vi "SUMMER SUNDAY BYTE[6].vi"() -> ()   [LabVIEW 2009]
uses:
  <vilib>/ULx/Create Channel.llb/ULx Create Channel (AI-Voltage-Basic).vi
  <vilib>/ULx/Create Channel.llb/ULx Create Channel (DO-Digital Output).vi
  <vilib>/ULx/Create Channel.llb/ULx Create Channel (DI-Digital Input).vi
  <vilib>/ULx/Write.llb/ULx Write (Digital Bool 1Line 1Point).vi
  <vilib>/ULx/Read.llb/ULx Read (Analog DBL 1Chan 1Samp).vi
  <vilib>/ULx/Read.llb/ULx Read (Digital 1D U8 NChan 1Samp).vi
  <vilib>/ULx/Read.llb/ULx Read (Digital Bool 1Line 1Point).vi
panel:
  out "BitValue":bool
  out "max value":u8
  out "POWER":bool
  out "data":dbl format="%_6g"
  out "ENERGY LEVEL":dbl(knob) scale=0.0..15.0
  out "Beam Pot":dbl format="%_6g"
  out "READY 2":bool
  out "DUMP":bool
  out "POWER":bool
  out "?":bool
  out "?":bool
  out "?":bool
  out "?":bool
  out "?":bool
  out "?":bool
  out "?":bool
  out "?":bool
  out "?":bool
  out "?":bool
  out "OPEN":bool
  out "CLOSED":bool
  out "READY":bool
  out "FAULT":bool
  out "MAGNET FORCE":dbl(slide) scale=0.0..10.0
  out "READY":bool
  out "TEMPERATURE":dbl(slide) scale=0.0..100.0
  in  "stop":bool
  out "?":bool
  out "?":bool
  out "?":bool
  out "?":bool
  out "FAULT":bool
  out "POWER":bool
  out "FLOW IN GPM":dbl(knob) scale=0.0..15.0
  # "USERS LAB AREA"
  # "BEAM STATUS"
  # "ROOM"
  # "XRAY"
  # "PUMP STATION"
  # "MAGNET STATUS"
  # "ORBIT"
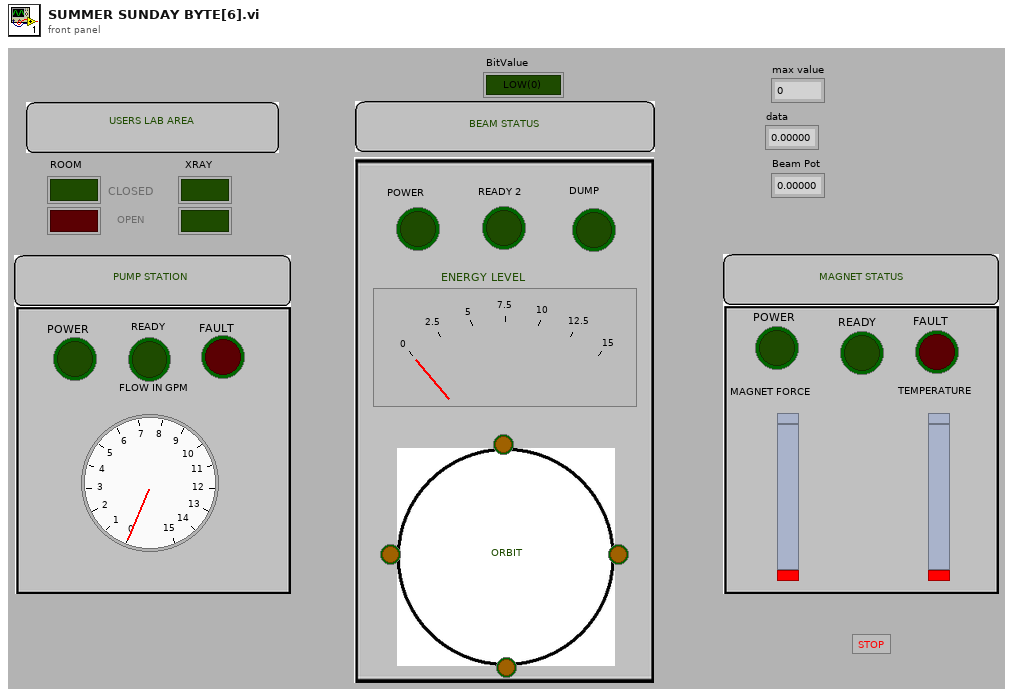
[diagram p1: front panel]
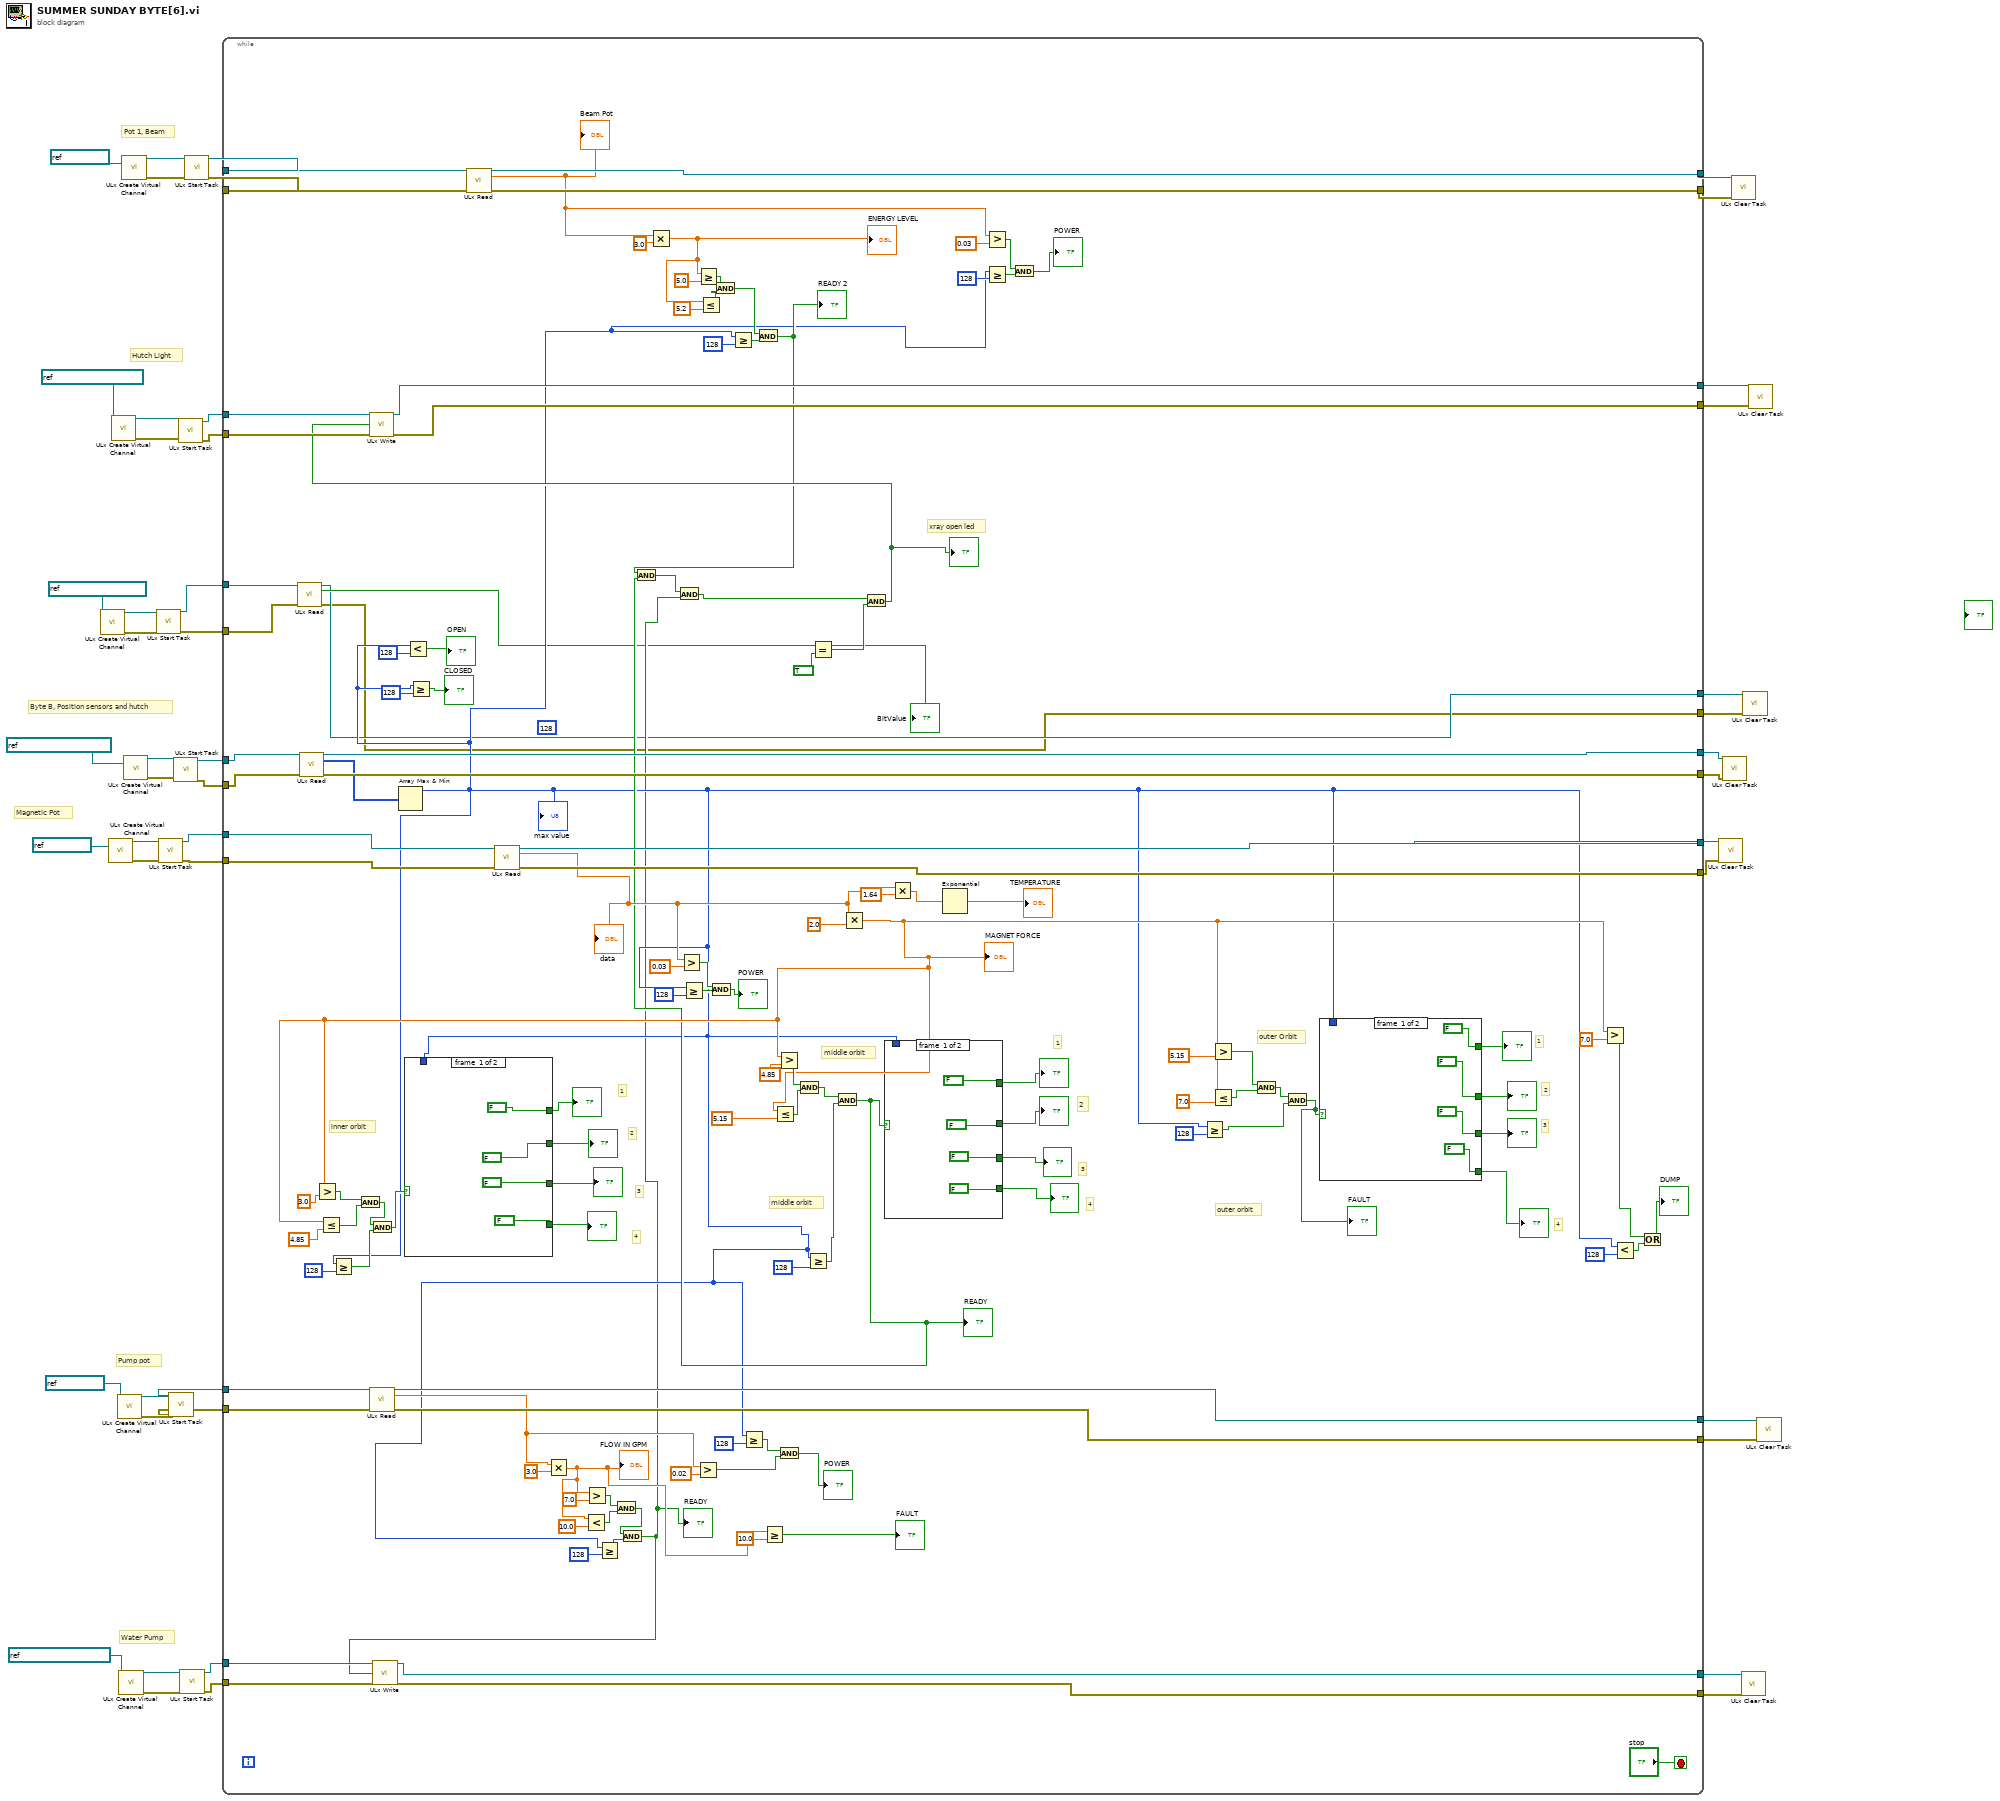
[diagram p0: block diagram]
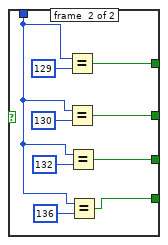
[diagram p2: hidden frame]
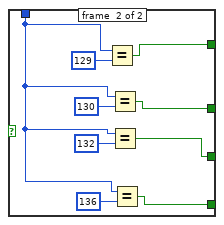
[diagram p3: hidden frame]
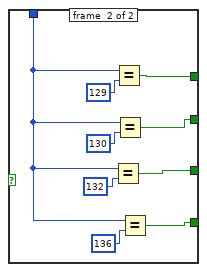
[diagram p4: hidden frame]
diagram:
  # "Water Pump"
  # "Pump pot"
  # "Hutch Light"
  # "Byte B, Position sensors and hutch"
  # "Magnetic Pot"
  # "Pot 1, Beam"
  n1 = call-poly <vilib>:"ULx Create Virtual Channel.vi"("lines"=refnum<k21> "Dev0/1stPortA/Di2") -> ("task out"=w7:refnum<k24>, "error out"=w6:errorcluster)  [unwired: 13 in]
  n2 = call-poly <vilib>:"ULx Create Virtual Channel.vi"("physical channels"=refnum<k21> "Dev0/Ai1") -> ("task out"=w43:refnum<k24>, "error out"=w42:errorcluster)  [unwired: 13 in]
  n3 = call-poly <vilib>:"ULx Create Virtual Channel.vi"("lines"=refnum<k21> "Dev0/1stPortA/Do0") -> ("task out"=w28:refnum<k24>, "error out"=w27:errorcluster)  [unwired: 13 in]
  n4 = call-poly <vilib>:"ULx Create Virtual Channel.vi"("physical channels"=refnum<k21> "Dev0/Ai2") -> ("task out"=w35:refnum<k24>, "error out"=w34:errorcluster)  [unwired: 13 in]
  n5 = call-poly <vilib>:"ULx Create Virtual Channel.vi"("lines"=refnum<k21> "Dev0/1stPortA/Do1") -> ("task out"=w14:refnum<k24>, "error out"=w13:errorcluster)  [unwired: 13 in]
  n6 = call-poly <vilib>:"ULx Create Virtual Channel.vi"("physical channels"=refnum<k21> "Dev0/Ai0") -> ("task out"=w49:refnum<k24>, "error out"=w48:errorcluster)  [unwired: 13 in]
  n7 = call-poly <vilib>:"ULx Create Virtual Channel.vi"("lines"=refnum<k21> "Dev0/1stPortB/Di0:7") -> ("task out"=w21:refnum<k24>, "error out"=w20:errorcluster)  [unwired: 13 in]
  n8 = call <vilib>:"ULx Start Task.vi"("task in"=w7, "error in"=w6) -> ("task out"=w4:refnum<k24>, "error out"=w3:errorcluster)  [unwired: 12 in]
  n9 = call <vilib>:"ULx Start Task.vi"("task in"=w43, "error in"=w42) -> ("task out"=w41:refnum<k24>, "error out"=w40:errorcluster)  [unwired: 12 in]
  n10 = call <vilib>:"ULx Start Task.vi"("task in"=w35, "error in"=w34) -> ("task out"=w33:refnum<k24>, "error out"=w32:errorcluster)  [unwired: 12 in]
  n11 = call <vilib>:"ULx Start Task.vi"("task in"=w21, "error in"=w20) -> ("task out"=w19:refnum<k24>, "error out"=w18:errorcluster)  [unwired: 12 in]
  n12 = call <vilib>:"ULx Start Task.vi"("task in"=w28, "error in"=w27) -> ("task out"=w25:refnum<k24>, "error out"=w24:errorcluster)  [unwired: 12 in]
  n13 = call <vilib>:"ULx Start Task.vi"("task in"=w14, "error in"=w13) -> ("task out"=w12:refnum<k24>, "error out"=w11:errorcluster)  [unwired: 12 in]
  n14 = call <vilib>:"ULx Start Task.vi"("task in"=w49, "error in"=w48) -> ("task out"=w47:refnum<k24>, "error out"=w46:errorcluster)  [unwired: 12 in]
  n15 = while {
    tunnel: w47 -> [w175]
    tunnel: w46 -> [w174]
    tunnel: [w173] -> w45
    tunnel: [w172] -> w44
    tunnel: w41 -> [w170]
    tunnel: w40 -> [w169]
    tunnel: [w168] -> w39
    tunnel: [w167] -> w38
    tunnel: w33 -> [w129]
    tunnel: w32 -> [w128]
    tunnel: [w127] -> w30
    tunnel: [w126] -> w29
    tunnel: w25 -> [w100]
    tunnel: w24 -> [w99]
    tunnel: [w98] -> w23
    tunnel: [w97] -> w22
    tunnel: w19 -> [w96]
    tunnel: w18 -> [w95]
    tunnel: [w94] -> w16
    tunnel: [w93] -> w15
    tunnel: w12 -> [w65]
    tunnel: w11 -> [w64]
    tunnel: [w63] -> w10
    tunnel: [w62] -> w9
    tunnel: w4 -> [w54]
    tunnel: w3 -> [w53]
    tunnel: [w51] -> w2
    tunnel: [w50] -> w1
    stop <- "stop" stop-if-true
    (unwired) i16 128 ("y")
    # "xray open led"
    # "outer Orbit"
    # "middle orbit"
    # "4"
    # "3"
    # "2"
    # "1"
    # "1"
    # "2"
    # "3"
    # "4"
    # "4"
    # "3"
    # "2"
    # "1"
    # "outer orbit"
    # "inner orbit"
    # "middle orbit"
    n16 = call-poly <vilib>:"ULx Read.vi"("task in"=w54, "error in"=w53) -> ("task out"=w51:refnum<k24>, "data"=w52:bool, "error out"=w50:errorcluster)  [unwired: 11 in]
    "BitValue" <- w52
    n17 = call-poly <vilib>:"ULx Read.vi"("task in"=w96, "error in"=w95) -> ("task out"=w94:refnum<k24>, "data"=w92:u8[], "error out"=w93:errorcluster)  [unwired: 11 in]
    n18 = call-poly <vilib>:"ULx Read.vi"("task in"=w129, "error in"=w128) -> ("task out"=w127:refnum<k24>, "data"=w122:dbl, "error out"=w126:errorcluster)  [unwired: 11 in]
    n19 = Array Max & Min(array=w92) -> (max value=w60:u8)  [unwired: 3 out]
    "max value" <- w60
    n20 = Greater Or Equal?(x=w60, y=i16 128) -> (x >= y?=w154:bool)
    n21 = Less?(x=w60, y=u8 128) -> (x < y?=→"OPEN":bool)
    n22 = Greater Or Equal?(x=w60, y=u8 128) -> (x >= y?=→"CLOSED":bool)
    n23 = call-poly <vilib>:"ULx Read.vi"("task in"=w175, "error in"=w174) -> ("task out"=w173:refnum<k24>, "data"=w101:dbl, "error out"=w172:errorcluster)  [unwired: 11 in]
    "Beam Pot" <- w101
    n24 = call-poly <vilib>:"ULx Read.vi"("task in"=w170, "error in"=w169) -> ("task out"=w168:refnum<k24>, "data"=w105:dbl, "error out"=w167:errorcluster)  [unwired: 11 in]
    "data" <- w105
    n25 = Multiply(x=w122, y=3.0) -> (x*y=w111:dbl)
    "FLOW IN GPM" <- w111
    n26 = Less?(x=w111, y=10.0) -> (x < y?=w109:bool)
    n27 = Greater?(x=w111, y=7.0) -> (0:w110:bool)
    n28 = Greater Or Equal?(x=w60, y=u8 128) -> (x >= y?=w80:bool)
    n29 = And(x=w110, y=w109) -> (x .and. y?=w78:bool)
    n30 = And(x=w78, y=w80) -> (x .and. y?=w55:bool)
    "READY" <- w55
    n31 = call-poly <vilib>:"ULx Write.vi"("task in"=w65, "data"=w55, "error in"=w64) -> ("task out"=w63:refnum<k24>, "error out"=w62:errorcluster)  [unwired: 10 in, 1 out]
    n32 = Multiply(x=w101, y=3.0) -> (x*y=w119:dbl)
    "ENERGY LEVEL" <- w119
    n33 = Greater?(x=w105, y=0.03) -> (0:w83:bool)
    n34 = Greater Or Equal?(x=w60, y=u8 128) -> (x >= y?=w82:bool)
    n35 = Greater?(x=w122, y=0.02) -> (0:w75:bool)
    n36 = Greater Or Equal?(x=w119, y=5.0) -> (x >= y?=w117:bool)
    n37 = Less Or Equal?(x=w119, y=5.2) -> (x <= y?=w116:bool)
    n38 = And(x=w83, y=w82) -> (x .and. y?=→"POWER":bool)
    n39 = And(x=w117, y=w116) -> (x .and. y?=w70:bool)
    n40 = Greater Or Equal?(x=w60, y=u8 128) -> (x >= y?=w72:bool)
    n41 = Greater Or Equal?(x=w60, y=u8 128) -> (x >= y?=w76:bool)
    n42 = And(x=w70, y=w72) -> (x .and. y?=w69:bool)
    "READY 2" <- w69
    n43 = Greater Or Equal?(x=w111, y=10.0) -> (x >= y?=→"FAULT":bool)
    n44 = And(x=w76, y=w75) -> (x .and. y?=→"POWER":bool)
    n45 = Greater Or Equal?(x=w60, y=i16 128) -> (x >= y?=w91:bool)
    n46 = Equal?(x=w52, y=TRUE) -> (x = y?=w85:bool)
    n47 = Multiply(x=w105, y=2.0) -> (x*y=w147:dbl)
    "MAGNET FORCE" <- w147
    n48 = Greater?(x=w147, y=3.0) -> (0:w163:bool)
    n49 = Less Or Equal?(x=w147, y=4.85) -> (x <= y?=w164:bool)
    n50 = And(x=w163, y=w164) -> (x .and. y?=w156:bool)
    n51 = And(x=w156, y=w154) -> (x .and. y?=w155:bool)
    n52 = case shown="True" w155 {
      tunnel: [FALSE w210] -> w132
      tunnel: [FALSE w209] -> w133
      tunnel: [FALSE w208] -> w130
      tunnel: [FALSE w207] -> w131
      tunnel: w60 -> [_ w215]
      frame #0 {
      }
      frame #1 {
        n53 = Equal?(x=w215, y=i16 132) -> (x = y?=w208:bool)
        n54 = Equal?(x=w215, y=i16 129) -> (x = y?=w210:bool)
        n55 = Equal?(x=w215, y=i16 130) -> (x = y?=w209:bool)
        n56 = Equal?(x=w215, y=i16 136) -> (x = y?=w207:bool)
      }
    }
    "?" <- w133
    "?" <- w130
    "?" <- w131
    "?" <- w132
    n57 = Less Or Equal?(x=w147, y=5.15) -> (x <= y?=w160:bool)
    n58 = Greater?(x=w147, y=4.85) -> (0:w161:bool)
    n59 = And(x=w161, y=w160) -> (x .and. y?=w153:bool)
    n60 = And(x=w153, y=w91) -> (x .and. y?=w89:bool)
    "READY" <- w89
    n61 = And(x=w69, y=w89) -> (x .and. y?=w88:bool)
    n62 = And(x=w88, y=w55) -> (x .and. y?=w86:bool)
    n63 = And(x=w86, y=w85) -> (x .and. y?=w84:bool)
    "?" <- w84
    n64 = call-poly <vilib>:"ULx Write.vi"("task in"=w100, "data"=w84, "error in"=w99) -> ("task out"=w98:refnum<k24>, "error out"=w97:errorcluster)  [unwired: 10 in, 1 out]
    n65 = case shown="True" w89 {
      tunnel: [FALSE w189] -> w142
      tunnel: [FALSE w188] -> w141
      tunnel: [FALSE w187] -> w140
      tunnel: [FALSE w186] -> w139
      tunnel: w60 -> [_ w185]
      frame #0 {
      }
      frame #1 {
        n66 = Equal?(x=w185, y=i16 129) -> (x = y?=w189:bool)
        n67 = Equal?(x=w185, y=i16 130) -> (x = y?=w188:bool)
        n68 = Equal?(x=w185, y=i16 132) -> (x = y?=w187:bool)
        n69 = Equal?(x=w185, y=i16 136) -> (x = y?=w186:bool)
      }
    }
    "?" <- w142
    "?" <- w141
    "?" <- w140
    "?" <- w139
    n70 = Multiply(x=w105, y=1.64) -> (x*y=w103:dbl)
    n71 = Exponential(1:w103) -> (0:→"TEMPERATURE":dbl)
    n72 = Greater?(x=w101, y=0.03) -> (0:w67:bool)
    n73 = Greater Or Equal?(x=w60, y=u8 128) -> (x >= y?=w73:bool)
    n74 = And(x=w67, y=w73) -> (x .and. y?=→"POWER":bool)
    n75 = Greater Or Equal?(x=w60, y=i16 128) -> (x >= y?=w137:bool)
    n76 = Greater?(x=w147, y=5.15) -> (0:w158:bool)
    n77 = Less Or Equal?(x=w147, y=7.0) -> (x <= y?=w157:bool)
    n78 = And(x=w158, y=w157) -> (x .and. y?=w146:bool)
    n79 = And(x=w146, y=w137) -> (x .and. y?=w106:bool)
    "FAULT" <- w106
    n80 = case shown="True" w106 {
      tunnel: [FALSE w194] -> w151
      tunnel: [FALSE w195] -> w150
      tunnel: [FALSE w196] -> w149
      tunnel: [FALSE w197] -> w148
      tunnel: w60 -> [_ w202]
      frame #0 {
      }
      frame #1 {
        n81 = Equal?(x=w202, y=i16 129) -> (x = y?=w197:bool)
        n82 = Equal?(x=w202, y=i16 130) -> (x = y?=w196:bool)
        n83 = Equal?(x=w202, y=i16 132) -> (x = y?=w195:bool)
        n84 = Equal?(x=w202, y=i16 136) -> (x = y?=w194:bool)
      }
    }
    "?" <- w148
    "?" <- w149
    "?" <- w150
    "?" <- w151
    n85 = Greater?(x=w147, y=7.0) -> (0:w107:bool)
    n86 = Less?(x=w60, y=i16 128) -> (x < y?=w134:bool)
    n87 = Or(x=w107, y=w134) -> (x .or. y?=→"DUMP":bool)
  }
  n88 = call <vilib>:"ULx Clear Task.vi"("task in"=w39, "error in"=w38) -> ()  [unwired: 13 in, 1 out]
  n89 = call <vilib>:"ULx Clear Task.vi"("task in"=w16, "error in"=w15) -> ()  [unwired: 13 in, 1 out]
  n90 = call <vilib>:"ULx Clear Task.vi"("task in"=w45, "error in"=w44) -> ()  [unwired: 13 in, 1 out]
  n91 = call <vilib>:"ULx Clear Task.vi"("task in"=w10, "error in"=w9) -> ()  [unwired: 13 in, 1 out]
  n92 = call <vilib>:"ULx Clear Task.vi"("task in"=w2, "error in"=w1) -> ()  [unwired: 13 in, 1 out]
  n93 = call <vilib>:"ULx Clear Task.vi"("task in"=w23, "error in"=w22) -> ()  [unwired: 13 in, 1 out]
  n94 = call <vilib>:"ULx Clear Task.vi"("task in"=w30, "error in"=w29) -> ()  [unwired: 13 in, 1 out]
